vi "findBG-index-IR-SD.vi"(1 "II channel in":u16[][](array[numeric]), 2 "I channel in":u16[][](array[numeric])) -> (0 "index BG":i32)   [LabVIEW 2015]
uses:
  globalVarSD.vi
panel:
  out "in":dbl[](graph) caption="Data Values"
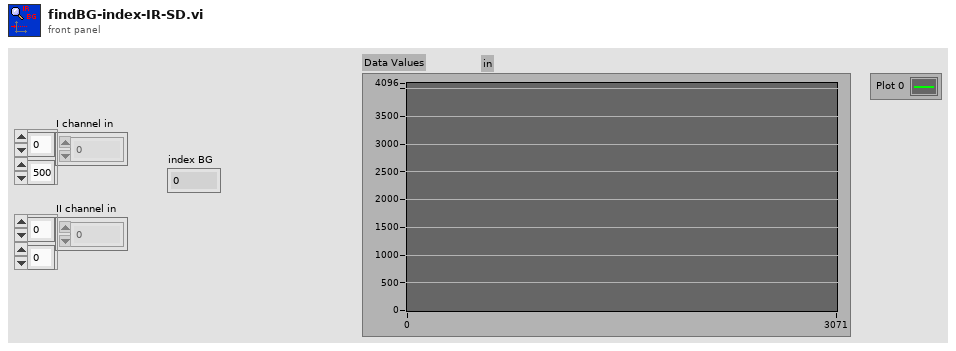
[diagram p1: front panel]
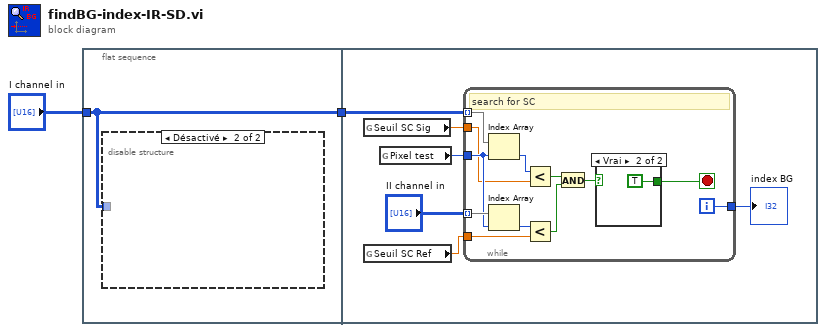
[diagram p0: block diagram]
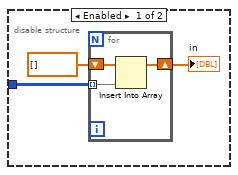
[diagram p2: hidden frame]
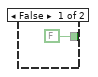
[diagram p3: hidden frame]
diagram:
  n1 = flat-sequence {
    tunnel: "I channel in" -> [w3]
    tunnel: [w3] -> w1
    tunnel: w1 -> [w10]
    frame #0 {
      n2 = disable-structure shown="Désactivé" {
        disable-tunnel: w3 -> [w4 _]
        frame Enabled {
          n3 = for {
            tunnel: w4 -> [w7] mode=indexing
            shift-right: [w8] -> w5
            shift-left: dbl[] [] ("tableau") -> [w9]
            n4 = Insert Into Array(array=w9, new element=w7) -> (w8:dbl[])  [unwired: 1 in]
          }
          "in" <- w5
        }
        frame Disabled {
        }
      }
    }
    frame #1 {
      n5 = global read "globalVarSD.vi" "Seuil SC Sig"() -> (w12:dbl)
      n6 = global read "globalVarSD.vi" "Seuil SC Ref"() -> (w13:dbl)
      n7 = global read "globalVarSD.vi" "Pixel test"() -> (w14:u32)
      n8 = while {
        tunnel: w10 -> [w25] mode=indexing
        tunnel: "II channel in" -> [w24] mode=indexing
        tunnel: w12 -> [w22]
        tunnel: w13 -> [w20]
        tunnel: w14 -> [w23]
        tunnel: [w17] -> w11
        i -> [w17]
        stop <- w18 stop-if-true
        # "search for SC"
        n9 = Index Array(array=w25, index=w23) -> (element=w21:u16)
        n10 = Index Array(array=w24, index=w23) -> (element=w19:u16)
        n11 = Less?(x=w21, y=w22) -> (x < y?=w27:bool)
        n12 = Less?(x=w19, y=w20) -> (x < y?=w26:bool)
        n13 = And(x=w27, y=w26) -> (x .and. y?=w16:bool)
        n14 = case shown="Vrai" w16 {
          tunnel: [FALSE TRUE] -> w18
          frame False {
          }
          frame True {
          }
        }
      }
      "index BG" <- w11
    }
  }
